vi "Update BuildSpec.vi"(7 "BuildSpec Sources":T1[](array[typedef])=[{"Source Library"="TimingDRV Engine.lvlib", "Source Folder"="Engine", "Apply Inclusion"=TRUE}, {"Source Library"="TimingDRV Shared.lvlib", "Source Folder"="Shared", "Apply Inclusion"=FALSE}, {"Source Library"="", "Source Folder"="NI VeriStand APIs", "Apply Inclusion"=FALSE}], 8 "error in (no error)":errorcluster, 10 "Target Build Spec":string, 11 "CD Build Tools in":refnum<class "Project Sync Tools.lvclass">) -> (0 "error out":errorcluster, 3 "CD Build Tools out":refnum<class "Project Sync Tools.lvclass">)   [LabVIEW 2019, in "Project Sync Tools.lvclass"]
uses:
  Project Sync Tools.lvclass
  TypeDefs/BuildSpec Source.ctl
  Project Sync Tools.lvclass/Project Sync Tools.ctl
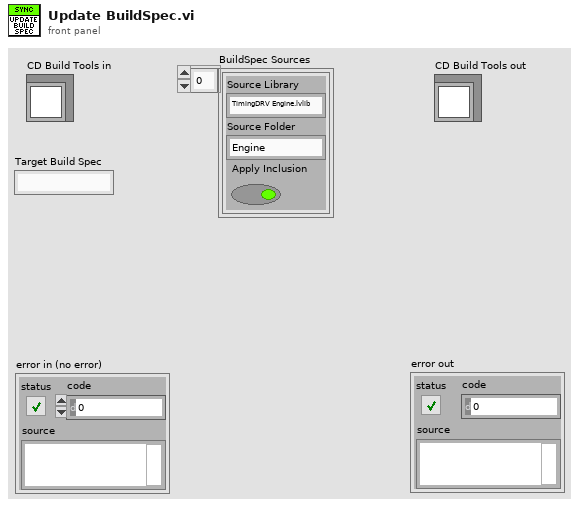
[diagram p1: front panel]
types:
  T1 = typedef "Project Sync Tools.lvclass/BuildSpec Source.ctl" = cluster{"Source Library":string, "Source Folder":string, "Apply Inclusion":bool}
  T2 = typedef "Project Sync Tools.lvclass/BuildSpec Parameters.ctl" = cluster{"BuildSpec Ref":refnum<vi>, "Target Name":string, "Build Spec Name":string, "Tags":string[], "Tag Values":variant[]}
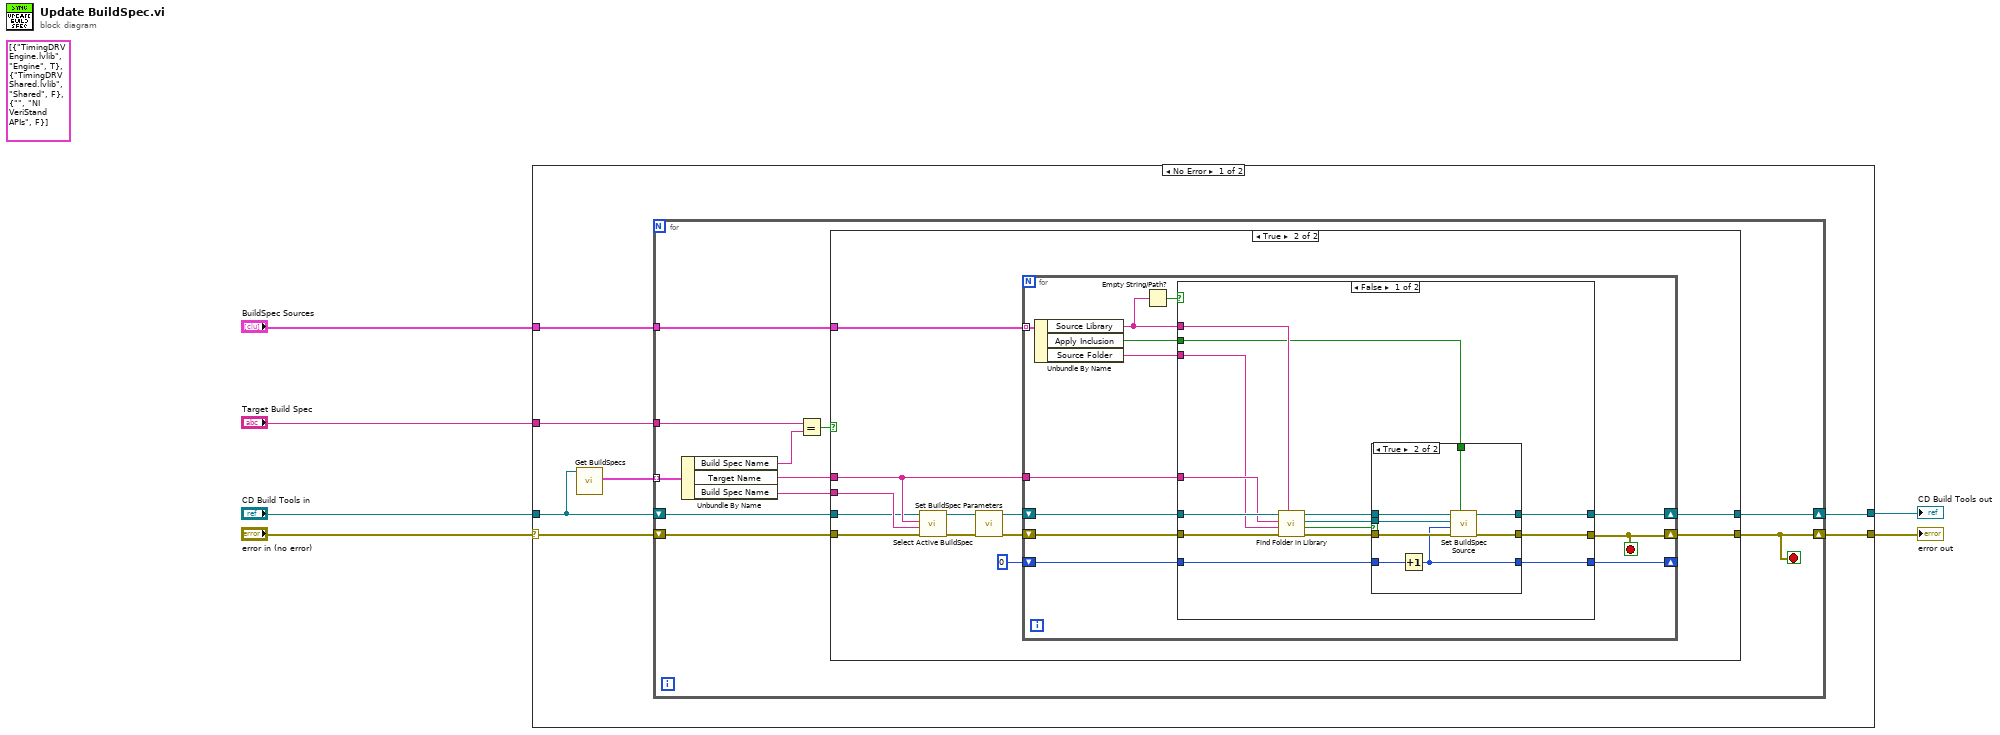
[diagram p0: block diagram]
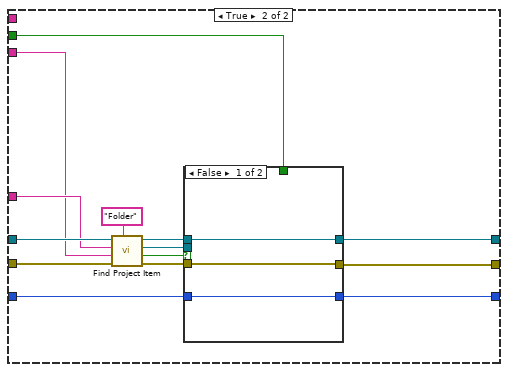
[diagram p4: hidden frame]
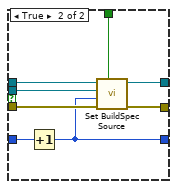
[diagram p5: hidden frame]
diagram:
  (unwired) T1[] [{"Source Library"="TimingDRV Engine.lvlib", "Source Folder"="Engine", "Apply Inclusion"=TRUE}, {"Source Library"="TimingDRV Shared.lvlib", "Source Folder"="Shared", "Apply Inclusion"=FALSE}, {"Source Library"="", "Source Folder"="NI VeriStand APIs", "Apply Inclusion"=FALSE}]
  n1 = case shown="No Error" "error in (no error)" {
    selector: "error in (no error)" -> [w11 w102]
    tunnel: "CD Build Tools in" -> [w12 w101]
    tunnel: [w10 w101] -> w5
    tunnel: [w9 w102] -> w3
    tunnel: "Target Build Spec" -> [w8 _]
    tunnel: "BuildSpec Sources" -> [w7 _]
    frame No Error {
      n2 = call "Get BuildSpecs.vi"("Project Sync Tools in"=w12) -> ("BuildSpecs"=w13:T2[])  [unwired: 9 in, 1 out]
      n3 = for {
        shift-right: [w19] -> w9
        shift-left: w11 -> [w24]
        shift-right: [w23] -> w10
        shift-left: w12 -> [w14]
        tunnel: w13 -> [w22] mode=indexing
        tunnel: w8 -> [w17]
        tunnel: w7 -> [w15]
        stop <- w19 stop-if-true
        n4 = Unbundle By Name(w22) -> ("Build Spec Name"=w18:string, "Target Name"=w21:string, "Build Spec Name"=w20:string)
        n5 = Equal?(x=w17, y=w18) -> (x = y?=w16:bool)
        n6 = case shown="True" w16 {
          tunnel: w24 -> [w26 w38]
          tunnel: [w25 w31] -> w23
          tunnel: w14 -> [w25 w29]
          tunnel: w21 -> [_ w33]
          tunnel: w20 -> [_ w36]
          tunnel: [w26 w30] -> w19
          tunnel: w15 -> [_ w35]
          frame False {
          }
          frame True {
            n7 = call "Select Active BuildSpec.vi"("error in (no error)"=w38, "Build Spec Name in"=w36, "Target Name in"=w33, "Project Sync Tools in"=w29) -> ("error out"=w37:errorcluster, "Project Sync Tools out"=w27:refnum<class "Project Sync Tools.lvclass">)  [unwired: 6 in]
            n8 = call "Set BuildSpec Parameters.vi"("Error In"=w37, "Project Sync Tools in"=w27) -> ("error out"=w34:errorcluster, "Project Sync Tools out"=w28:refnum<class "Project Sync Tools.lvclass">)  [unwired: 8 in]
            n9 = for {
              tunnel: w35 -> [w50] mode=indexing
              shift-right: [w40] -> w31
              shift-left: w28 -> [w46]
              tunnel: w33 -> [w45]
              shift-right: [w41] -> _
              shift-left: 0 ("Source Index") -> [w42]
              shift-right: [w39] -> w30
              shift-left: w34 -> [w47]
              stop <- w39 stop-if-true
              n10 = Unbundle By Name(w50) -> ("Source Library"=w48:string, "Apply Inclusion"=w43:bool, "Source Folder"=w44:string)
              n11 = Empty String/Path?(string/path=w48) -> (empty?=w49:bool)
              n12 = case shown="False" w49 {
                tunnel: w48 -> [w62 _]
                tunnel: w47 -> [w60 w89]
                tunnel: w46 -> [w64 w88]
                tunnel: w45 -> [w63 w86]
                tunnel: w44 -> [w61 w83]
                tunnel: w43 -> [w53 w82]
                tunnel: w42 -> [w55 w79]
                tunnel: [w52 w78] -> w41
                tunnel: [w54 w77] -> w40
                tunnel: [w51 w76] -> w39
                frame False {
                  n13 = call "Find Folder in Library.vi"("Library Name"=w62, "error in (no error)"=w60, "Folder Name"=w61, "Target Name"=w63, "Project Sync Tools in"=w64) -> ("error out"=w59:errorcluster, "Found?"=w56:bool, "Folder Ref out"=w57:refnum<vi>, "Project Sync Tools out"=w58:refnum<class "Project Sync Tools.lvclass">)  [unwired: 3 in]
                  n14 = case shown="True" w56 {
                    tunnel: w59 -> [w66 w75]
                    tunnel: w57 -> [_ w74]
                    tunnel: w58 -> [w67 w73]
                    tunnel: [w67 w72] -> w54
                    tunnel: [w66 w71] -> w51
                    tunnel: w55 -> [w65 w70]
                    tunnel: [w65 w69] -> w52
                    tunnel: w53 -> [_ w68]
                    frame False {
                    }
                    frame True {
                      n15 = Increment(x=w70) -> (x+1=w69:i32)
                      n16 = call "Set BuildSpec Source.vi"("Apply Inclusion ?"=w68, "Error In"=w75, "Source Index"=w69, "Source Item in"=w74, "Project Sync Tools in"=w73) -> ("error out"=w71:errorcluster, "Project Sync Tools out"=w72:refnum<class "Project Sync Tools.lvclass">)  [unwired: 5 in]
                    }
                  }
                }
                frame True {
                  n17 = call "Find Project Item.vi"("Type"="Folder", "error in (no error)"=w89, "Item Name"=w83, "Target Name"=w86, "Project Sync Tools in"=w88) -> ("error out"=w85:errorcluster, "Found ?"=w81:bool, "ProjectItem out"=w80:refnum<vi>, "Project Sync Tools out"=w84:refnum<class "Project Sync Tools.lvclass">)  [unwired: 3 in]
                  n18 = case shown="False" w81 {
                    tunnel: w85 -> [w90 w100]
                    tunnel: w84 -> [w91 w99]
                    tunnel: w82 -> [_ w98]
                    tunnel: w80 -> [_ w97]
                    tunnel: [w90 w96] -> w76
                    tunnel: [w91 w95] -> w77
                    tunnel: w79 -> [w92 w94]
                    tunnel: [w92 w93] -> w78
                    frame False {
                    }
                    frame True {
                      n19 = Increment(x=w94) -> (x+1=w93:i32)
                      n20 = call "Set BuildSpec Source.vi"("Apply Inclusion ?"=w98, "Error In"=w100, "Source Index"=w93, "Source Item in"=w97, "Project Sync Tools in"=w99) -> ("error out"=w96:errorcluster, "Project Sync Tools out"=w95:refnum<class "Project Sync Tools.lvclass">)  [unwired: 5 in]
                    }
                  }
                }
              }
            }
          }
        }
      }
    }
    frame Error {
    }
  }
  "CD Build Tools out" <- w5
  "error out" <- w3
